vi "Get Sample Rate.vi"(8 "error in (no error)":errorcluster, 11 "RTL-SDR in":refnum<class "Session.lvclass">) -> (0 "error out":errorcluster, 2 "Sample Rate":u32 format="%#.12p", 3 "RTL-SDR out":refnum<class "Session.lvclass">)   [LabVIEW 2021, in "RTL-SDR.lvlib" / "Session.lvclass"]
uses:
  Session.lvclass
  Session.lvclass/Session.ctl
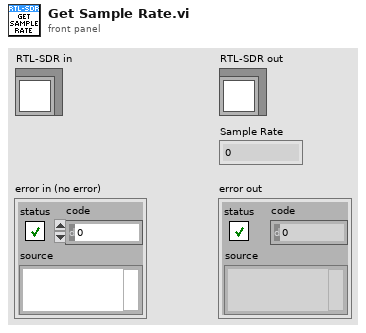
[diagram p1: front panel]
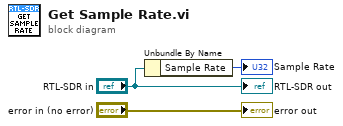
[diagram p0: block diagram]
diagram:
  n1 = Unbundle By Name("RTL-SDR in") -> ("Sample Rate"=→"Sample Rate":u32)
  "error out" <- "error in (no error)"
  "RTL-SDR out" <- "RTL-SDR in"
